vi "scanFrontPanel.vi"(8 "error in (no error)":errorcluster, 9 "index":i16, 10 "ScriptEventList":refnum<class "ScriptEventList.lvclass">, 11 "ScanCreator in":refnum<class "ScanCreator.lvclass">) -> (0 "error out":errorcluster, 1 "cancelled":bool, 2 "scriptListArray":refnum<class "ScriptEventList.lvclass">[](array[class]), 3 "ScanCreator out":refnum<class "ScanCreator.lvclass">, 4 "scanType":string, 5 "Values":string[](array[string]))   [LabVIEW 2009, in "Views.lvlib" / "ScriptEditor.lvlib" / "ScanCreator.lvclass"]
uses:
  ScanCreator.lvclass
  Tools/Scripting/ScriptingEvent/ScriptEventList/ScriptEventList.lvclass
  ScanCreator.lvclass/ScanCreator.ctl
panel:
  in  "Cancel":bool
  in  "ok":bool
  in  "Delay All?":bool=TRUE
  in  "Number of Steps":i16
  in  "EndValue":dbl format="%#_8g"
  in  "StartValue":dbl format="%#.8g"
  in  "Scan Type":u16(ring) items=["Time", "Time Difference", "Start Value", "End Value", "Step Value", "Ramp Time"]
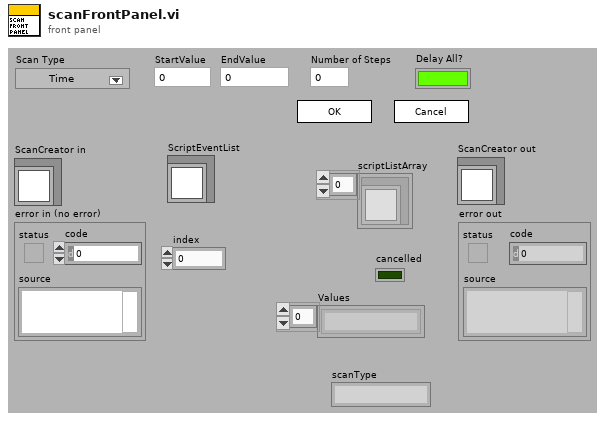
[diagram p1: front panel]
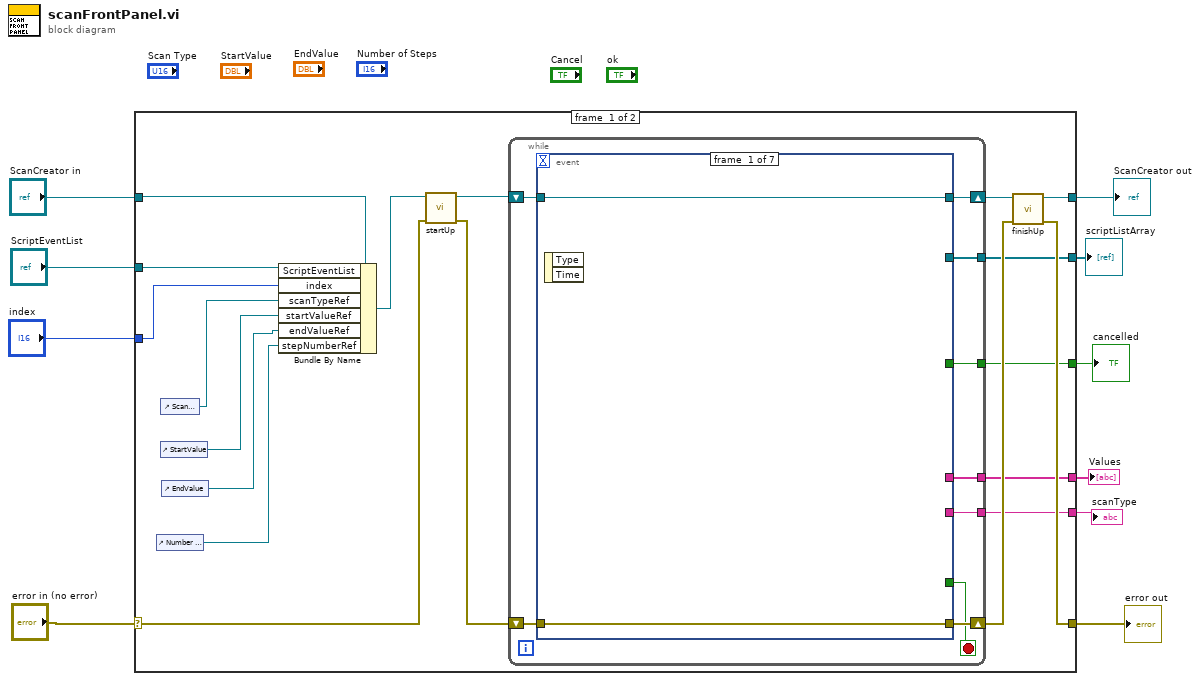
[diagram p0: block diagram]
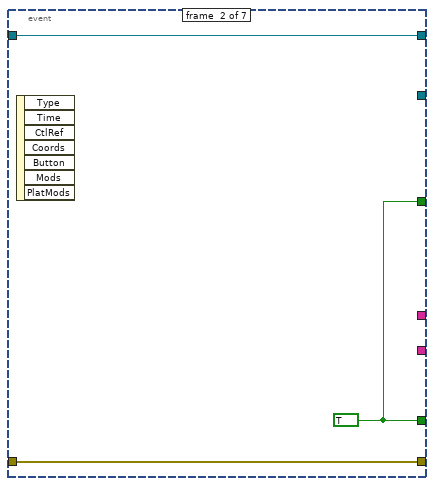
[diagram p2: hidden frame]
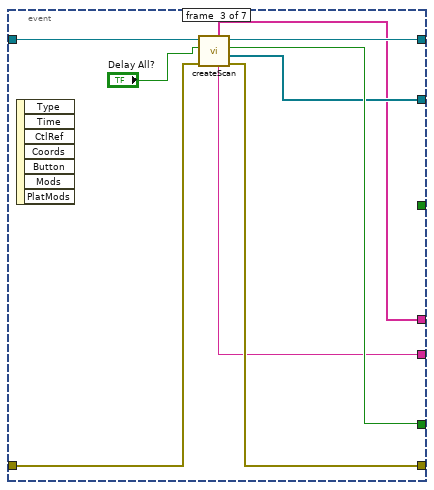
[diagram p3: hidden frame]
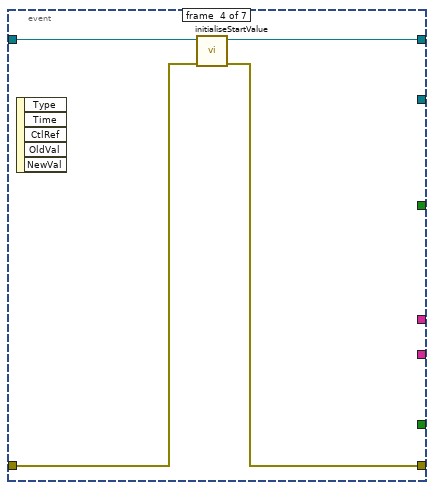
[diagram p4: hidden frame]
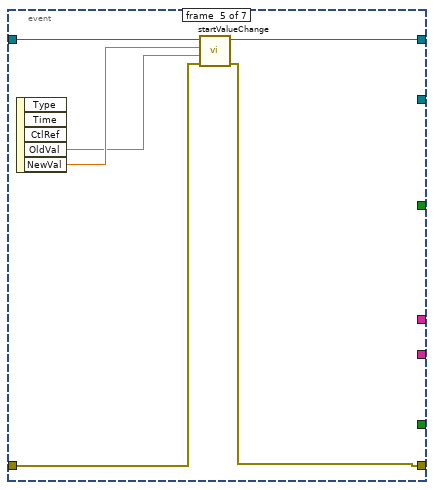
[diagram p5: hidden frame]
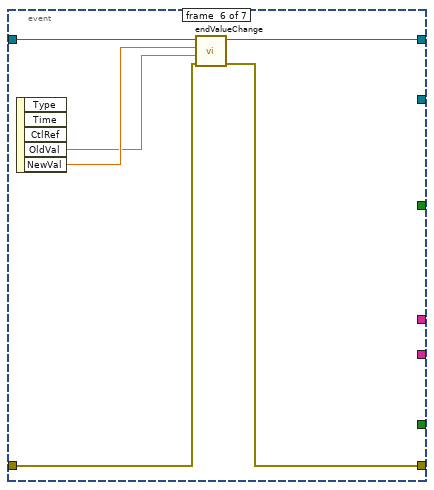
[diagram p6: hidden frame]
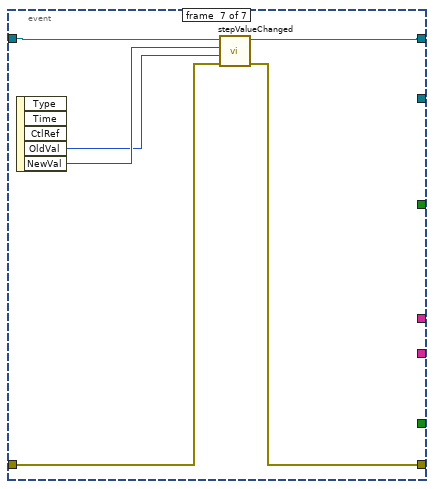
[diagram p7: hidden frame]
diagram:
  n1 = case shown="No Error" "error in (no error)" {
    selector: "error in (no error)" -> [w28 w76]
    tunnel: [w23 w76] -> w9
    tunnel: [w25 w75] -> w7
    tunnel: "ScanCreator in" -> [w18 w75]
    tunnel: "ScriptEventList" -> [w22 _]
    tunnel: "index" -> [w21 _]
    tunnel: [w16 _] -> w4
    tunnel: [w15 _] -> w3
    tunnel: [w14 _] -> w2
    tunnel: [w13 _] -> w1
    frame #0 {
      n2 = control-ref of="Number of Steps"() -> (w19:refnum<vi>)
      n3 = control-ref of="Scan Type"() -> (w11:refnum<vi>)
      n4 = control-ref of="StartValue"() -> (w20:refnum<vi>)
      n5 = control-ref of="EndValue"() -> (w12:refnum<vi>)
      n6 = Bundle By Name(cluster=w18, "ScriptEventList"=w22, "index"=w21, "scanTypeRef"=w11, "startValueRef"=w20, "endValueRef"=w12, "stepNumberRef"=w19) -> (w17:refnum<class "ScanCreator.lvclass">)
      n7 = call "startUp.vi"("error in (no error)"=w28, "ScanCreator in"=w17) -> ("error out"=w27:errorcluster, "ScanCreator out"=w29:refnum<class "ScanCreator.lvclass">)  [unwired: 8 in]
      n8 = while {
        shift-right: [w38] -> w24
        shift-left: w27 -> [w37]
        shift-right: [w36] -> w26
        shift-left: w29 -> [w35]
        tunnel: [w33] -> w16
        tunnel: [w32] -> w15
        tunnel: [w31] -> w14
        tunnel: [w30] -> w13
        stop <- w34 stop-if-true
        n9 = event shown="[5] \"EndValue\": Value Change" {
          selector: _ -> [_ _ _ _ _ _ _]
          dyn-events: _ -> [_ _ _ _ _ _ _]
          timeout: _ -> [_ _ _ _ _ _ _]
          tunnel: [w40 w42 w50 w53 w59 w66 w69] -> w38
          tunnel: w37 -> [w40 w42 w51 w54 w60 w65 w70]
          tunnel: [w39 w43 w49 w55 w61 w67 w73] -> w36
          tunnel: w35 -> [w39 w43 w52 w56 w62 w68 w74]
          tunnel: [_ w41 w48 _ _ _ _] -> w34
          tunnel: [_ _ w46 _ _ _ _] -> w33
          tunnel: [_ w41 _ _ _ _ _] -> w32
          tunnel: [_ _ w45 _ _ _ _] -> w31
          tunnel: [_ _ w44 _ _ _ _] -> w30
          event #0 {
            n10 = event-data() -> ()  [unwired: 1 in, 2 out]
          }
          event #1 {
            w41 = TRUE
            n11 = event-data() -> ()  [unwired: 1 in, 7 out]
          }
          event #2 {
            n12 = event-data() -> ()  [unwired: 1 in, 7 out]
            n13 = call "createScan.vi"("error in (no error)"=w51, "delayAll"="Delay All?", "ScanCreator in"=w52) -> ("error out"=w50:errorcluster, "scriptListArray"=w46:refnum<class "ScriptEventList.lvclass">[], "close"=w48:bool, "ScanCreator out"=w49:refnum<class "ScanCreator.lvclass">, "scanType"=w44:string, "Values"=w45:string[])  [unwired: 3 in]
          }
          event #3 {
            n14 = event-data() -> ()  [unwired: 1 in, 5 out]
            n15 = call "initialiseStartValue.vi"("error in (no error)"=w54, "ScanCreator in"=w56) -> ("error out"=w53:errorcluster, "ScanCreator out"=w55:refnum<class "ScanCreator.lvclass">)  [unwired: 8 in]
          }
          event #4 {
            n16 = event-data() -> ("OldVal"=w57:dbl, "NewVal"=w58:dbl)  [unwired: 1 in, 3 out]
            n17 = call "startValueChange.vi"("error in (no error)"=w60, "oldValue"=w57, "newValue"=w58, "ScanCreator in"=w62) -> ("error out"=w59:errorcluster, "ScanCreator out"=w61:refnum<class "ScanCreator.lvclass">)  [unwired: 6 in]
          }
          event #5 {
            n18 = event-data() -> ("OldVal"=w63:dbl, "NewVal"=w64:dbl)  [unwired: 1 in, 3 out]
            n19 = call "endValueChange.vi"("error in (no error)"=w65, "oldValue"=w63, "newValue"=w64, "ScanCreator in"=w68) -> ("error out"=w66:errorcluster, "ScanCreator out"=w67:refnum<class "ScanCreator.lvclass">)  [unwired: 6 in]
          }
          event #6 {
            n20 = event-data() -> ("OldVal"=w71:i16, "NewVal"=w72:i16)  [unwired: 1 in, 3 out]
            n21 = call "stepValueChanged.vi"("error in (no error)"=w70, "oldValue"=w71, "newValue"=w72, "ScanCreator in"=w74) -> ("error out"=w69:errorcluster, "ScanCreator out"=w73:refnum<class "ScanCreator.lvclass">)  [unwired: 5 in, 1 out]
          }
        }
      }
      n22 = call "finishUp.vi"("error in (no error)"=w24, "ScanCreator in"=w26) -> ("error out"=w23:errorcluster, "ScanCreator out"=w25:refnum<class "ScanCreator.lvclass">)  [unwired: 8 in]
    }
    frame #1 {
    }
  }
  "error out" <- w9
  "ScanCreator out" <- w7
  "scriptListArray" <- w4
  "cancelled" <- w3
  "Values" <- w2
  "scanType" <- w1
